vi "ask_poly.vi"   [LabVIEW 2020, in "agent_simple_qa.lvclass"]
uses:
  agent_simple_qa.lvclass
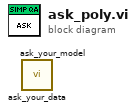
[diagram p0: block diagram]
diagram:
  n1 = call "ask_your_data.vi"() -> ()  [unwired: 9 in, 3 out]
  n2 = call "ask_your_model.vi"() -> ()  [unwired: 9 in, 3 out]
